vi "Hide Dynamic Tangent.vi"(8 "error in (no error)":errorcluster, 10 "Residuals":bool, 11 "WaveformGraph in":refnum<vi>) -> (0 "error out":errorcluster, 3 "WaveformGraph out":refnum<vi>)   [LabVIEW 2013, in "main.lvlib"]
uses:
  main.lvlib
  Controls/Enum Variables.ctl
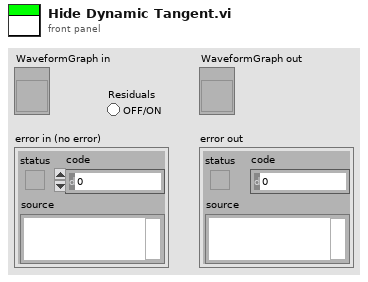
[diagram p1: front panel]
types:
  T1 = typedef "main.lvlib/Enum Variables.ctl" = enum16{"SetAcqFilter", "GetAcqFilter", "Set Filter", "Get Filter", "Set Height", "Get Height", "Set Recorded Height", "Get Recorded Height", "Set Blue Pressure", "Get Blue Pressure", "Set Red Pressure", "Get Red Pressure", "Init", "Reset Pressure", "Set Red Cursors", "Get Red Cursors", "Set Blue Cursors", "Get Blue Cursors", "Set Language", "Get Language", "Set Active Graphs", "Get ActiveGraphs", "Set Method", "Get Method", "Set Encryption", "Get Encryption", "Set ExcelVersion", "Get ExcelVersion", "Set DICOM Avail", "Get DICOM Avail", "Set DICOM Encode", "Get DICOM Encode", "Set JournalExport", "Get JournalExport", "Set Sequence", "Get Sequence", "Set DAQ Connected", "Get DAQ Connected", "Set Current Graph", "Get Current Graph", "Set General Settings", "Get Hyphenation", "Set Arm Calc Method", "Get Arm Calc Method", "Set Dicom Tags", "Get Dicom Tags", "Set BT Serial", "Get BT Serial", "Set BT Accepted Serials", "Get BT Accepted Serials", "Get BT License", "Set BT License"}
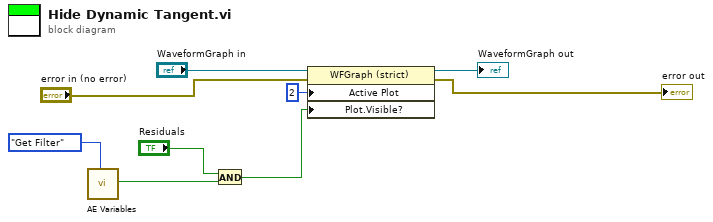
[diagram p0: block diagram]
diagram:
  n1 = call "AE Variables.vi"("Action"=Enum_Variables."Get Filter") -> ("BooleanOut"=w3:bool)  [unwired: 11 in, 7 out]
  n2 = And(x="Residuals", y=w3) -> (x .and. y?=w1:bool)
  n3 = property class="WFGraph (strict)"(reference="WaveformGraph in", error in="error in (no error)", "Active Plot"=u32 2, "Plot.Visible?"=w1) -> (reference out=→"WaveformGraph out":refnum<vi>, error out=→"error out":errorcluster)
